vi "IoT Logger Main.vi"() -> ()   [LabVIEW 2019]
uses:
  <vilib>/Utility/miscctls.llb/LVDateTimeRec.ctl
  SubVI/UI/Controls/Pages Tab.ctl
  SubVI/UI/Controls/Home Sensor Heading.ctl
  SubVI/UI/Controls/Buttons/Download Logs.ctl
  SubVI/UI/Controls/Connecting Ring.ctl
  SubVI/UI/Controls/Buttons/Real-time Data.ctl
  SubVI/UI/Controls/Log Row.ctl
  SubVI/UI/Controls/Log Row Download State Indicator.ctl
  SubVI/UI/Controls/Log.ctl
  SubVI/UI/Controls/Log State.ctl
  SubVI/Comms/State Controller/Controls/Comms Loop States.ctl
  SubVI/Messages/Typedefs/Message.ctl
  SubVI/Messages/Typedefs/Sensor Types.ctl
  SubVI/Messages/Typedefs/Message Types.ctl
  SubVI/Application Support/Stop Button/SubVI/Set Stop Button Status.vi
  SubVI/Application Support/Stop Button/SubVI/Get Stop Button Status.vi
  SubVI/Messages/Message Globals.vi
  <userlib>/_OpenG.lib/comparison/comparison.llb/Boolean Changed__ogtk.vi
panel:
  out "Pages":T1
  out "Connecting":T2
  out "Waiting Text":string
  in  "Comissioning":bool
  in  "Real-Time Button":T3
  out "Home Sensor Heading":T4 {"Slide" scale=0.0..100.0; "Free Space" format="%.1f%"}
  in  "Download Button":T5
  out "Log Row 6":T6 {"Download Progress" format="%d%"; "Log Progress" scale=0.0..100.0}
  out "Log Row 5":T6 {"Download Progress" format="%d%"; "Log Progress" scale=0.0..100.0}
  out "Log Row 4":T6 {"Download Progress" format="%d%"; "Log Progress" scale=0.0..100.0}
  out "Log Row 3":T6 {"Download Progress" format="%d%"; "Log Progress" scale=0.0..100.0}
  out "Log Row 2":T6 {"Download Progress" format="%d%"; "Log Progress" scale=0.0..100.0}
  out "Log Row 1":T6 {"Download Progress" format="%d%"; "Log Progress" scale=0.0..100.0}
  out "All Logs Heading":T4 {"Slide" scale=0.0..100.0; "Free Space" format="%.1f%"}
  out "Real-Time Home Heading":T4 {"Slide" scale=0.0..100.0; "Free Space" format="%.1f%"}
  in  "Commissioning Tab":T8(tab)
  in  "Get Log List":bool
  in  "Delete Log File":bool
  in  "Log File to delete":string
  in  "Log File Name":string
  in  "Get Log File":bool
  out "File Size":u32
  in  "Get Log File Size":bool
  out "File Transfer Progress":u32(slide) scale=0.0..54.0
  out "Logs Out":T9[](array[typedef])
  in  "Get SD Card Info":bool
  out "Used SD Card Space (mb)":sgl
  out "Sensor Errors":string[](array[string])
  in  "Send":bool
  in  "Data":u8[](array[numeric])
  in  "Message ID":u8
  in  "Sensor Type":u8
  in  "Payload Length":u8
  out "Turbidity 3":dbl
  out "Turbidity 2":dbl
  out "Turbidity 1":dbl
  out "Turbidity Temp":dbl
  out "Current Measurments":string
  in  "Get Measurements":bool
  in  "Decimal Places":u32=2
  in  "Get RTC Time":bool
  in  "New time":timestamp
  out "Current RTC Time":T11
  out "Logging Period":u32
  in  "Set Logging Period":bool
  in  "Logging Period ms":i32
  in  "Get Logging Period":bool
  out "App Name":string
  in  "Connect":bool
  out "Raw ADC":u32
  out "Battery Voltage":sgl
  in  "Get Battery Info":bool
  in  "Set WiFi Details":bool
  in  "Get WiFi Details":bool
  out "Current WiFi SSID":string
  out "Current WiFi Password":string
  in  "New WiFi Password":string
  in  "New WiFi SSID":string
  out "Heartbeat":bool
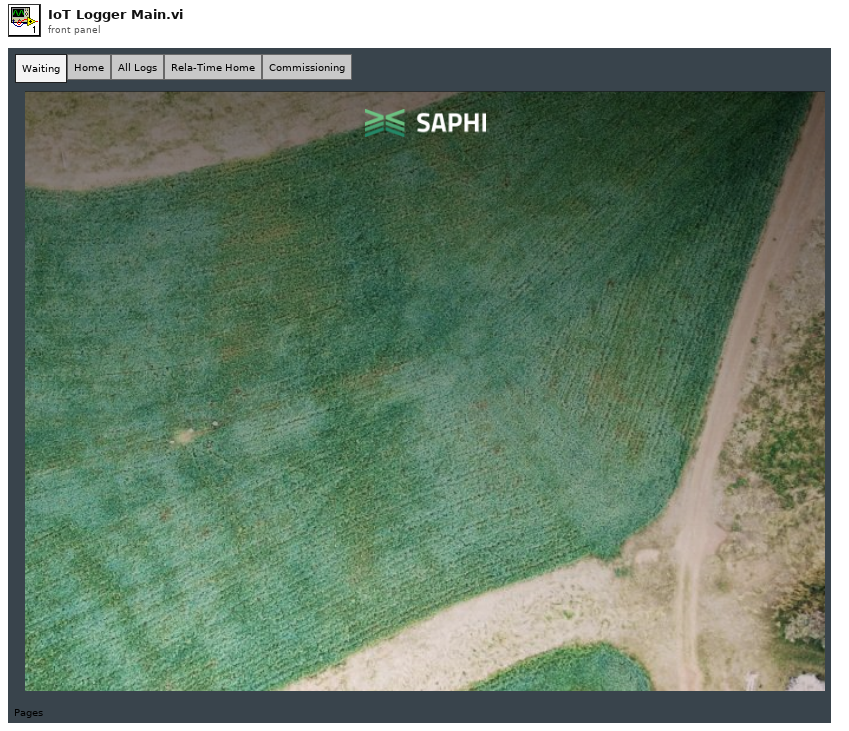
[diagram p1: front panel]
types:
  T1 = typedef "Pages Tab.ctl" = enum32{"Waiting", "Home", "All Logs", "Rela-Time Home", "Commissioning"}
  T2 = typedef "Connecting Ring.ctl" = u16
  T3 = typedef "Real-time Data.ctl" = bool
  T4 = typedef "Home Sensor Heading.ctl" = cluster{"Sensor Name":string, "Free Space":dbl, "Slide":dbl}
  T5 = typedef "Download Logs.ctl" = bool
  T6 = typedef "Log Row.ctl" = cluster{"Day":string, "Date":string, "Log Row Download":T7, "Download Progress":u8, "Log Progress":dbl}
  T7 = typedef "Log Row Download State Indicator.ctl" = u16
  T8 = enum32{"Log Functions", "SD Card Info", "Errors", "Custom Message", "Current Measurements", "RTC", "Logging Period", "Connect", "Batt", "WiFi"}
  T9 = typedef "Log.ctl" = cluster{"Name":string, "Download Percentage":dbl, "Log State":T10}
  T10 = typedef "Log State.ctl" = enum16{"New", "Downloading", "Downloaded"}
  T11 = typedef "LVDateTimeRec.ctl" = cluster{"fractional second":dbl, "second":i32, "minute":i32, "hour":i32, "day of month":i32, "month":i32, "year":i32, "day of week":i32, "day of year":i32, "DST":i32}
  T12 = typedef "Comms Loop States.ctl" = enum16{"Initalise", "User Event", "HEART_BEAT", "SEND_LOG_FILE_NAME", "Clear Log File Names", "SEND_LOG_FILE_CHUNK", "SEND_LOG_FILE_SIZE", "SEND_SD_CARD_INFO", "SEND_BATTERY_INFO", "SEND_LOGGING_PERIOD", "SEND_RTC_TIME", "SEND_CURRENT_MEASUREMENTS", "ERROR_MSG", "Clear Error Messages", "Send Message", "Idle", "Sensor Connected", "Sensor Disconnected", "Set Page Displayed", "Set Connected Sensor Type", "UI: Update Sensor Type", "UI: Update Log List", "Reset Log File Transfer", "SEND_WIFI_DETAILS"}
  T13 = typedef "Message.ctl" = cluster{"Payload Size":u8, "Sequence Number":u8, "Sensor Type":T14, "Message Types":T15, "Data":u8[]}
  T14 = typedef "Sensor Types.ctl" = enum16{"APP", "TURBIDITY", "PH"}
  T15 = typedef "Message Types.ctl" = enum16{"HEART_BEAT", "CONNECT", "GET_CURRENT_MEASUREMENTS", "GET_LOG_FILE", "SEND_LOG_FILE_SIZE", "SEND_LOG_FILE_CHUNK", "GET_LOGGING_PERIOD", "SET_LOGGING_PERIOD", "SEND_SD_CARD_INFO", "GET_LOGS_LIST", "SEND_LOG_FILE_NAME", "SEND_LOGGING_PERIOD", "GET_RTC_TIME", "SET_RTC_TIME", "SEND_RTC_TIME", "SEND_CURRENT_MEASUREMENTS", "DELETE_LOG_FILE", "GET_SD_CARD_INFO", "GET_BATTERY_INFO", "SEND_BATTERY_INFO", "GET_LOG_FILE_SIZE", "SET_WIFI_SSID", "SET_WIFI_PASSWORD", "GET_WIFI_DETAILS", "SEND_WIFI_DETAILS", "ERROR_MSG"}
  T16 = enum16{"open", "replace", "create", "open or create", "replace or create", "replace or create with confirmation"}
  T17 = typedef "eventvkey.ctl" = enum16{"ASCII", "Enter", "Return", "Shift", "Ctrl", "Alt", "Cmd", "Opt", "Caps", "NumLock", "Clear", "Break", "Up", "Down", "Left", "Right", "Insert", "Delete", "Home", "End", "PageUp", "PageDown", "Escape", "Help", "Pause", "ScrollLock", "F1", "F2", "F3", "F4", "F5", "F6", "F7", "F8", "F9", "F10", "F11", "F12", "F13", "F14", "F15", "F16", "F17", "F18", "F19", "F20", "F21", "F22", "F23", "F24", "Play", "VolumeUp", "VolumeDown", "Mute", "Two Byte Char"}
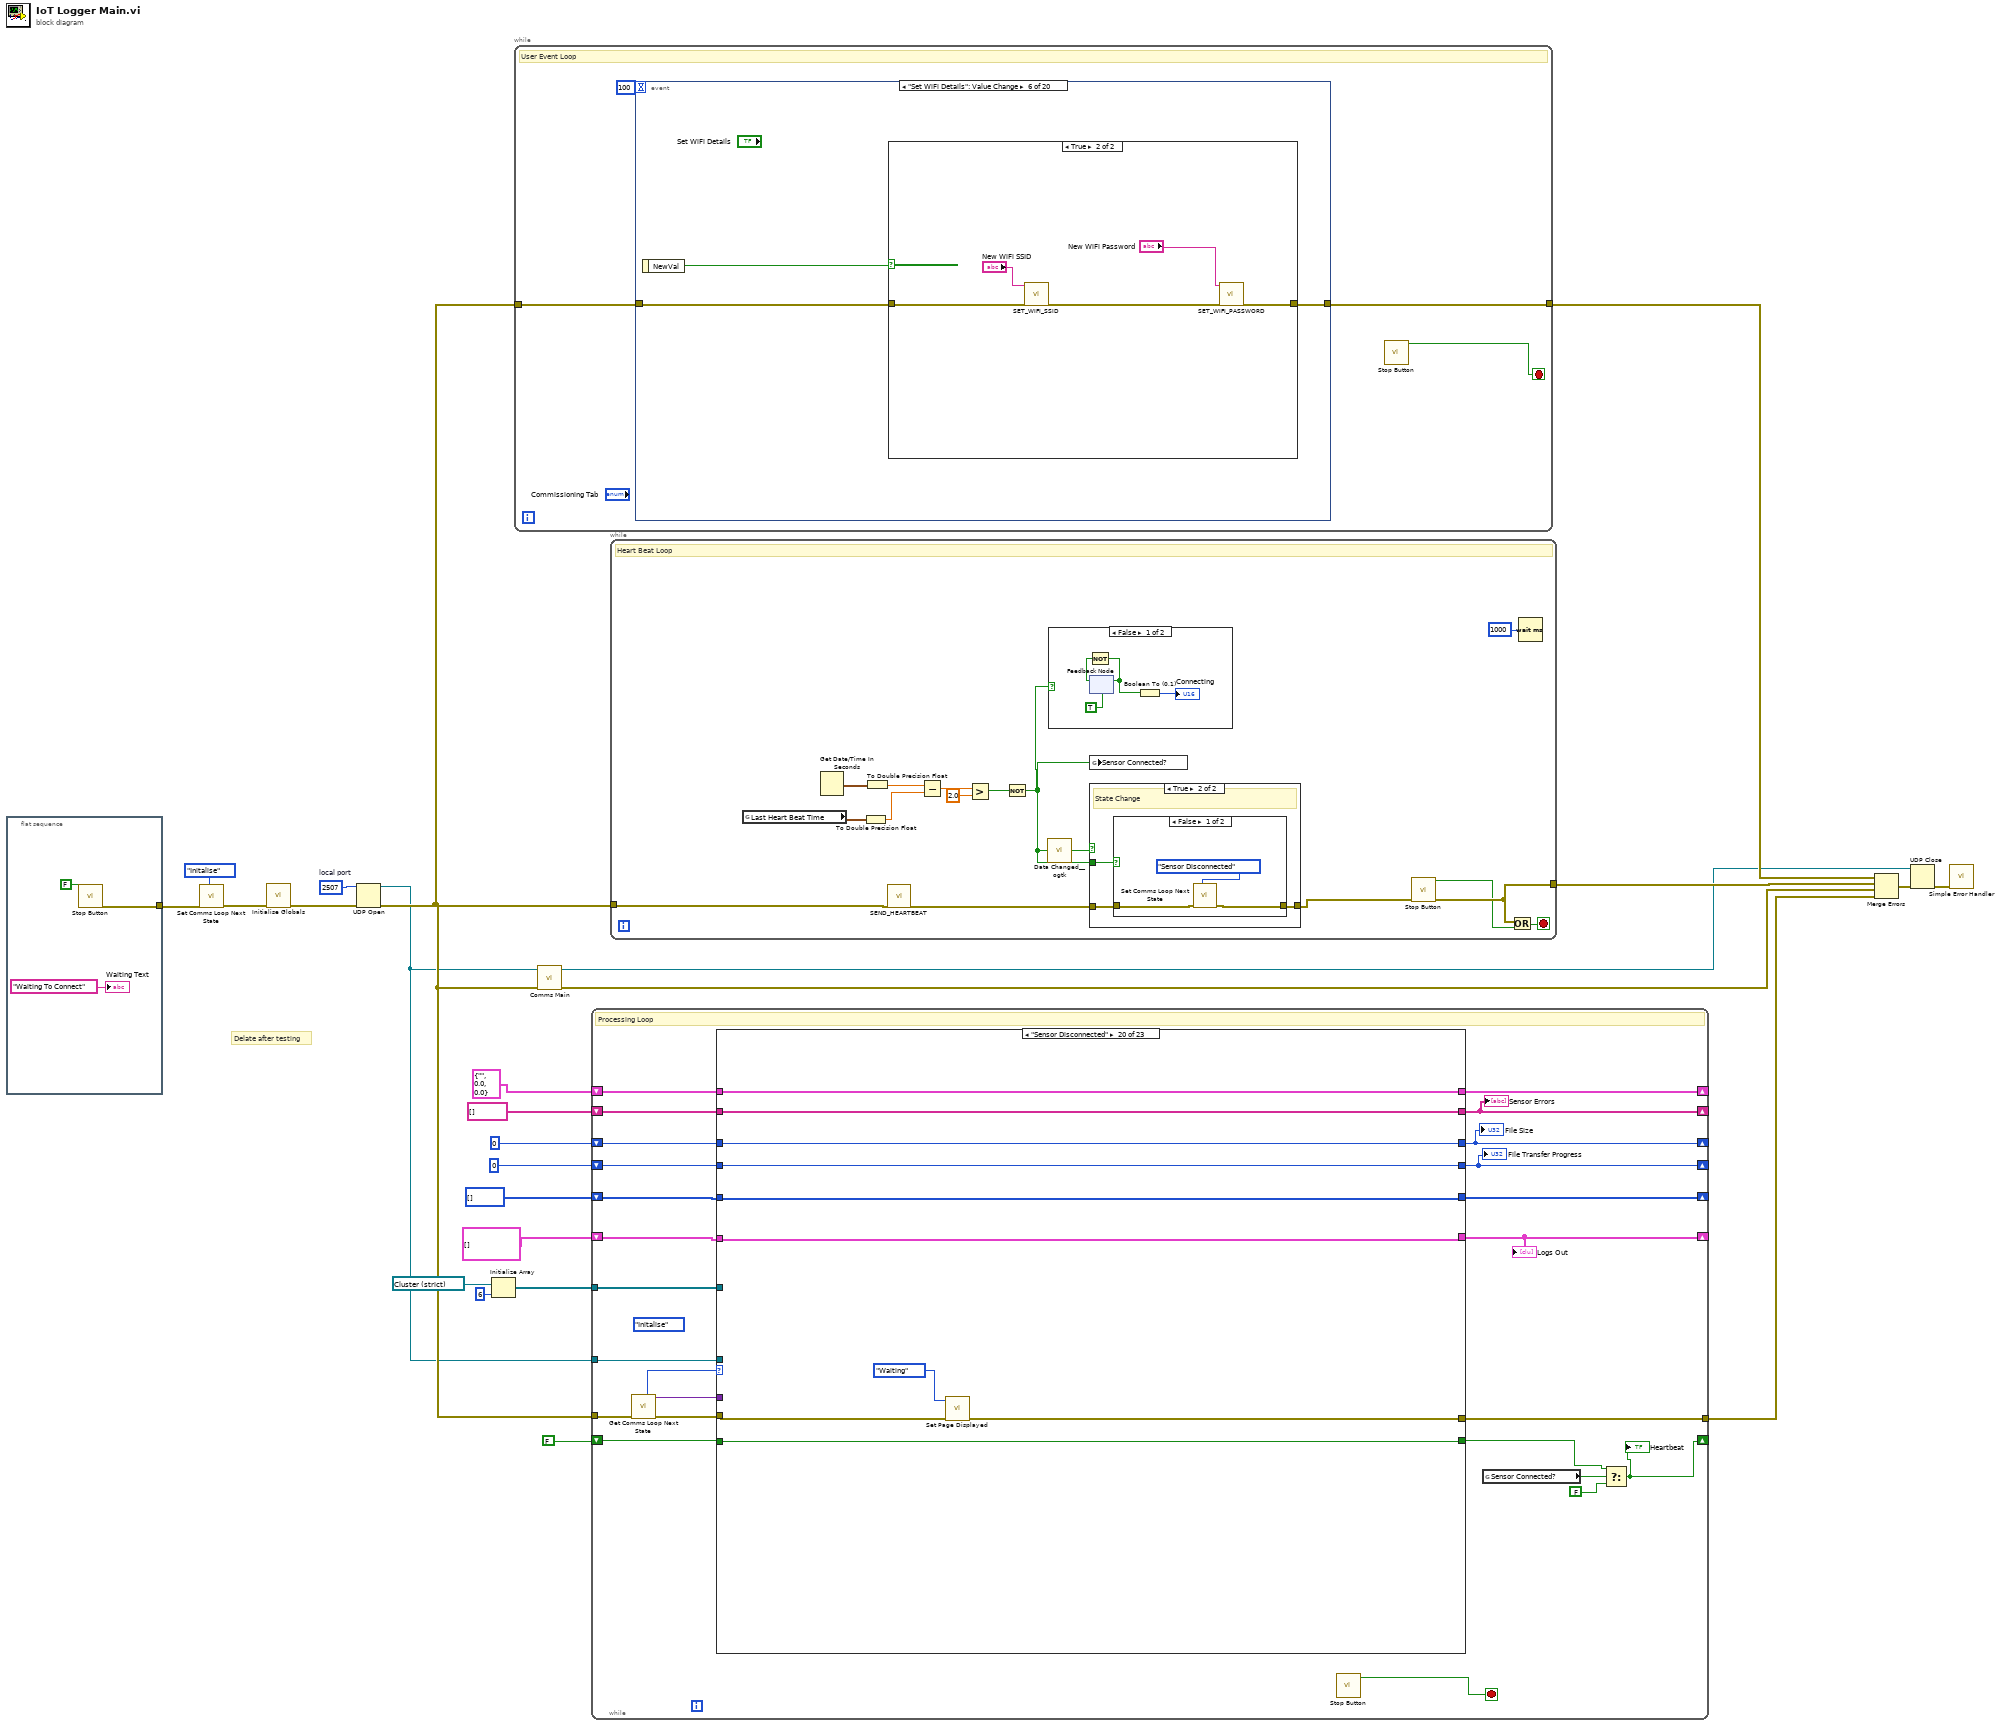
[diagram p0: block diagram]
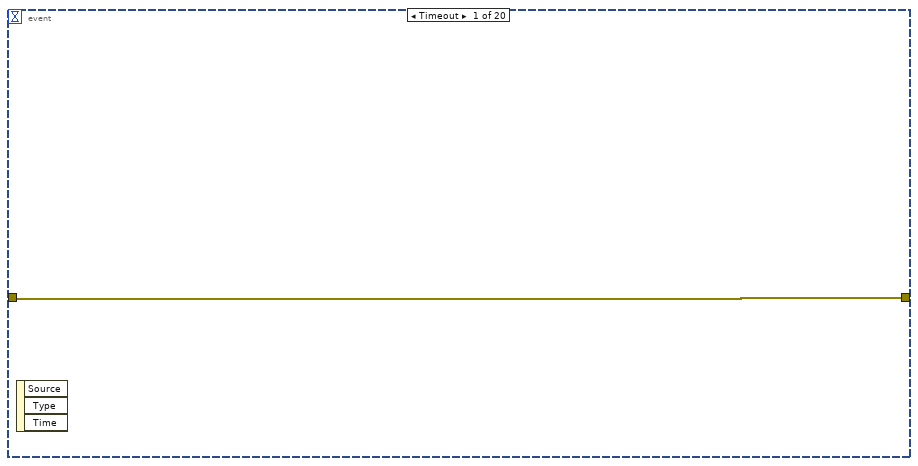
[diagram p2: hidden frame]
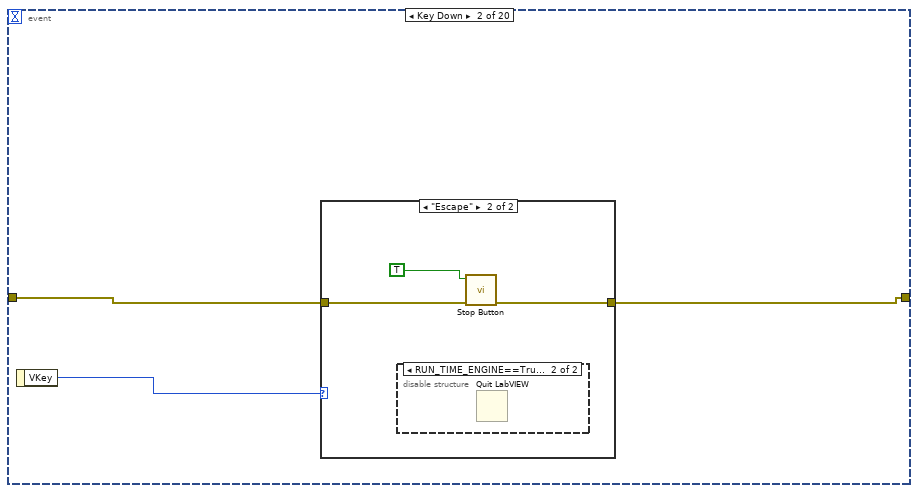
[diagram p3: hidden frame]
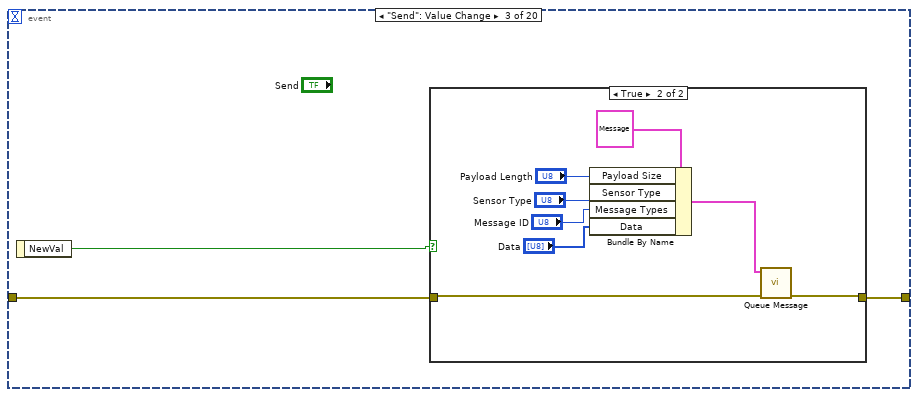
[diagram p6: hidden frame]
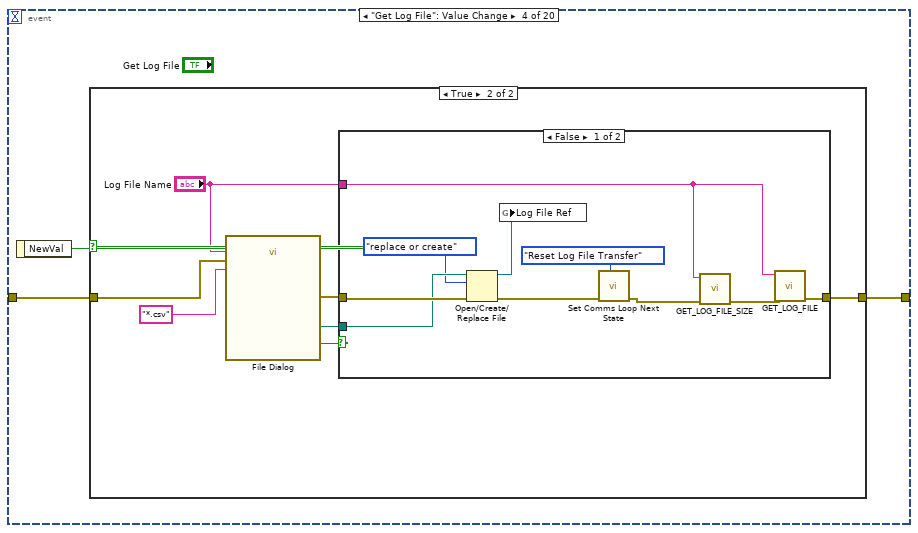
[diagram p8: hidden frame]
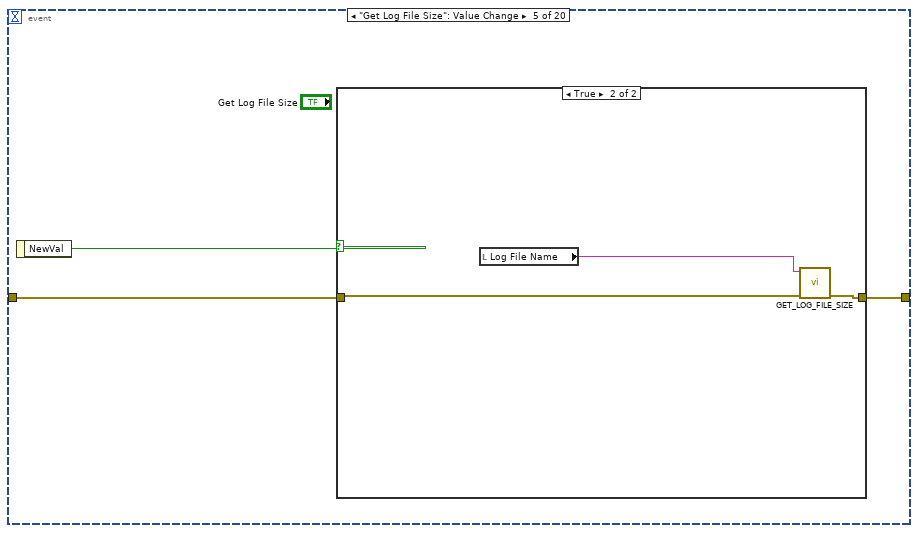
[diagram p11: hidden frame]
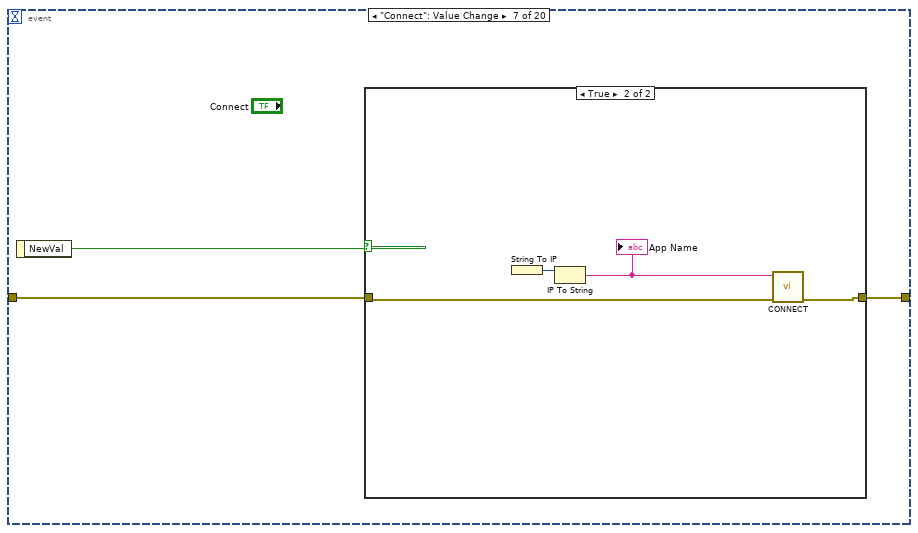
[diagram p14: hidden frame]
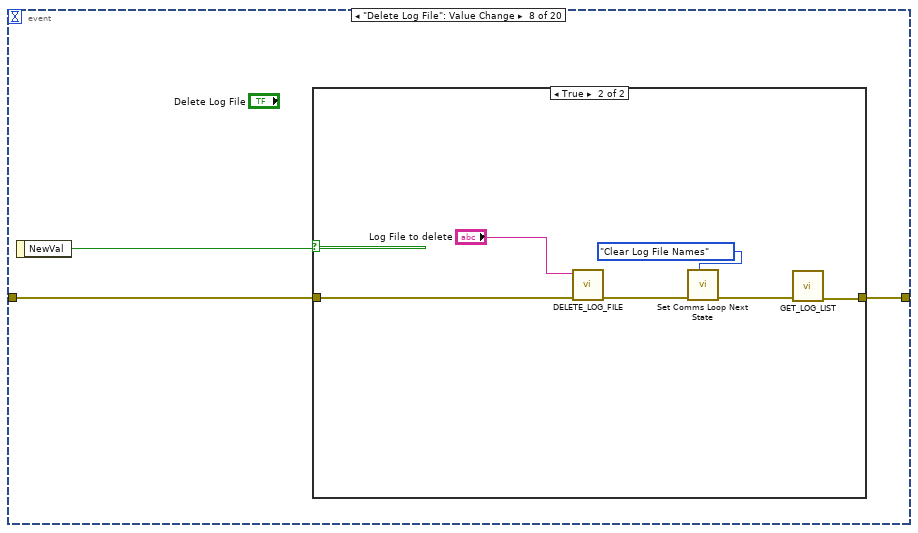
[diagram p16: hidden frame]
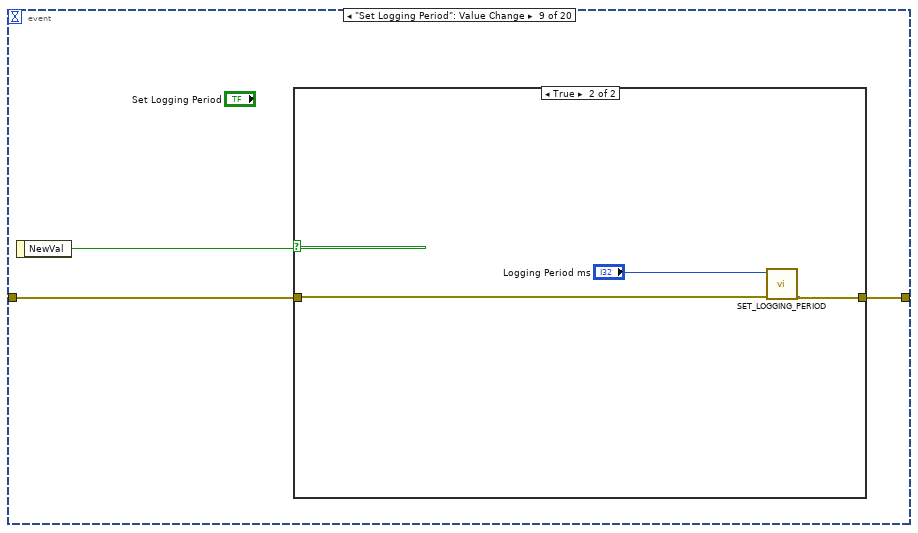
[diagram p18: hidden frame]
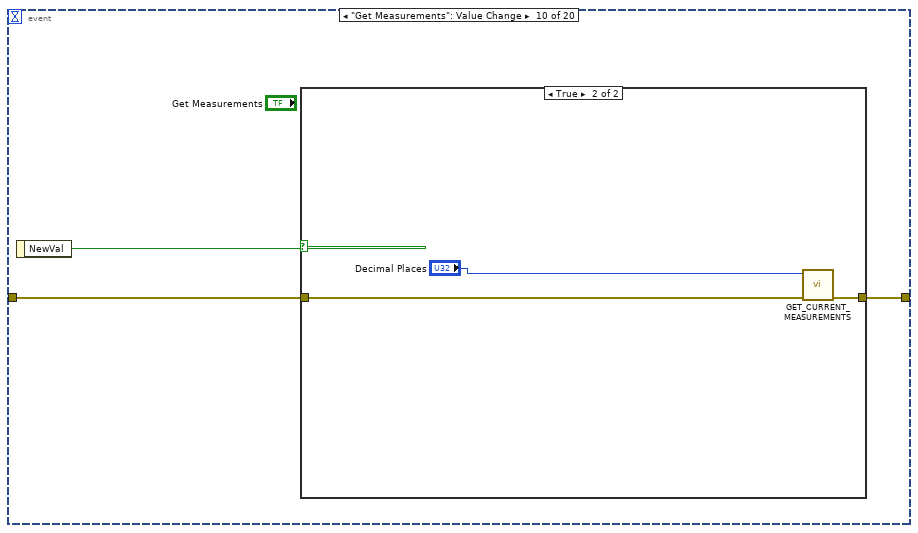
[diagram p20: hidden frame]
diagram:
  w24 = u16 2507  # local port
  # "Delate after testing"
  n1 = flat-sequence {
    tunnel: [w26] -> w5
    frame #0 {
      n2 = call-poly "Stop Button.vi"("Stop Button"=FALSE) -> ("Error Out"=w26:errorcluster)  [unwired: 10 in]
      "Waiting Text" <- "Waiting To Connect" ("Waiting Text")
    }
  }
  n3 = call "Set Comms Loop Next State.vi"("Command"=Comms_Loop_States."Initalise", "error in (no error)"=w5) -> ("error out"=w8:errorcluster)  [unwired: 9 in]
  n4 = call "Initialise Globals.vi"("error in (no error)"=w8) -> ("error out"=w7:errorcluster)  [unwired: 10 in]
  n5 = UDP Open(8:w7, 11:w24) -> (port=w9:refnum<k16>, 0:w19:errorcluster)  [unwired: 3 in, 1 out]
  n6 = Initialize Array(refnum<vi> refnum ("Log Row 1"), 6 ("dimension size")) -> (w2:refnum<vi>[])
  n7 = while {
    tunnel: w19 -> [w30]
    tunnel: [w29] -> w13
    stop <- w31 stop-if-true
    # "User Event Loop"
    n8 = event shown="[5] \"Set WiFi Details\": Value Change" {
      selector: _ -> [_ _ _ _ _ _ _ _ _ _ _ _ _ _ _ _ _ _ _ _]
      dyn-events: _ -> [_ _ _ _ _ _ _ _ _ _ _ _ _ _ _ _ _ _ _ _]
      timeout: 100 -> [_ _ _ _ _ _ _ _ _ _ _ _ _ _ _ _ _ _ _ _]
      tunnel: w30 -> [w32 w34 w41 w53 w75 w82 w91 w99 w109 w116 w123 w129 w135 w141 w147 w155 w161 w165 w168 w171]
      tunnel: [w32 w33 w40 w52 w74 w81 w90 w98 w108 w115 w122 w128 w134 w140 w146 w154 w162 w164 w167 w170] -> w29
      event Timeout {
        n9 = event-data() -> ()  [unwired: 1 in, 3 out]
      }
      event Key Down {
        n10 = event-data() -> ("VKey"=w35:T17)  [unwired: 1 in]
        n11 = case shown="\"Escape\"" w35 {
          tunnel: w34 -> [w36 w38]
          tunnel: [w36 w37] -> w33
          frame "ASCII", Default {
          }
          frame "Escape" {
            n12 = disable-structure shown="RUN_TIME_ENGINE==True" {
              frame condition #0 (active) {
              }
              frame condition #1 {
                n13 = Quit LabVIEW() -> ()  [unwired: 1 in]
              }
            }
            n14 = call-poly "Stop Button.vi"("Error In"=w38, "Stop Button"=TRUE ("Stop Simulator")) -> ("Error Out"=w37:errorcluster)  [unwired: 9 in]
          }
        }
      }
      event "Send": Value Change {
        n15 = event-data() -> ("NewVal"=w42:bool)  [unwired: 1 in]
        n16 = case shown="True" w42 {
          tunnel: w41 -> [w43 w44]
          tunnel: [w43 w51] -> w40
          frame False {
          }
          frame True {
            n17 = Bundle By Name(cluster=T13 {"Payload Size"=0, "Sequence Number"=0, "Sensor Type"=enum."APP", "Message Types"=enum."HEART_BEAT", "Data"=[]} ("Message"), "Payload Size"="Payload Length", "Sensor Type"="Sensor Type", "Message Types"="Message ID", "Data"="Data") -> (w45:T13)
            n18 = call "Queue Message.vi"("error in (no error)"=w44, "Message"=w45) -> ("error out"=w51:errorcluster)  [unwired: 9 in]
          }
        }
      }
      event "Get Log File": Value Change {
        n19 = event-data() -> ("NewVal"=w54:bool)  [unwired: 1 in]
        n20 = case shown="True" w54 {
          tunnel: w53 -> [w55 w61]
          tunnel: [w55 w62] -> w52
          frame False {
          }
          frame True {
            n21 = call "File Dialog"("default name"="Log File Name", "error in"=w61, "pattern (all files)"="*.csv") -> ("selected path"=w59:path, "cancelled"=w60:bool, "error out"=w58:errorcluster)  [unwired: 9 in, 1 out]
            n22 = case shown="False" w60 {
              tunnel: [w68 w73] -> w62
              tunnel: w58 -> [w72 w73]
              tunnel: w59 -> [w71 _]
              tunnel: "Log File Name" -> [w64 _]
              frame False {
                n23 = Open/Create/Replace File(file path (use dialog)=w71, error in=w72, operation (0:open)=T16."replace or create") -> (refnum out=w70:refnum<file>, error out=w67:errorcluster)  [unwired: 3 in, 1 out]
                n24 = global write "Message Globals.vi" "Log File Ref"(w70) -> ()
                n25 = call "Set Comms Loop Next State.vi"("Command"=Comms_Loop_States."Reset Log File Transfer", "error in (no error)"=w67) -> ("error out"=w65:errorcluster)  [unwired: 9 in]
                n26 = call "GET_LOG_FILE_SIZE.vi"("error in (no error)"=w65, "Log File Name"=w64) -> ("error out"=w66:errorcluster)  [unwired: 9 in]
                n27 = call "GET_LOG_FILE.vi"("error in (no error)"=w66, "Log File Name"=w64) -> ("error out"=w68:errorcluster)  [unwired: 9 in]
              }
              frame True {
              }
            }
          }
        }
      }
      event "Get Log File Size": Value Change {
        n28 = event-data() -> ("NewVal"=w76:bool)  [unwired: 1 in]
        n29 = case shown="True" w76 {
          tunnel: w75 -> [w77 w78]
          tunnel: [w77 w80] -> w74
          frame False {
          }
          frame True {
            n30 = local read "Log File Name"() -> (w79:string)
            n31 = call "GET_LOG_FILE_SIZE.vi"("error in (no error)"=w78, "Log File Name"=w79) -> ("error out"=w80:errorcluster)  [unwired: 9 in]
          }
        }
      }
      event "Set WiFi Details": Value Change {
        n32 = event-data() -> ("NewVal"=w83:bool)  [unwired: 1 in]
        n33 = case shown="True" w83 {
          tunnel: w82 -> [w84 w87]
          tunnel: [w84 w89] -> w81
          frame False {
          }
          frame True {
            n34 = call "SET_WIFI_SSID.vi"("error in (no error)"=w87, "New Wifi SSID"="New WiFi SSID") -> ("error out"=w86:errorcluster)  [unwired: 9 in]
            n35 = call "SET_WIFI_PASSWORD.vi"("error in (no error)"=w86, "New Wifi Password"="New WiFi Password") -> ("error out"=w89:errorcluster)  [unwired: 9 in]
          }
        }
      }
      event "Connect": Value Change {
        n36 = event-data() -> ("NewVal"=w92:bool)  [unwired: 1 in]
        n37 = case shown="True" w92 {
          tunnel: w91 -> [w93 w95]
          tunnel: [w93 w96] -> w90
          frame False {
          }
          frame True {
            n38 = String To IP() -> (0:w97:u32)  [unwired: 1 in]
            n39 = IP To String(2:w97) -> (0:w94:string)  [unwired: 1 in]
            "App Name" <- w94
            n40 = call "CONNECT.vi"("error in (no error)"=w95, "Local IP Address"=w94) -> ("error out"=w96:errorcluster)  [unwired: 9 in]
          }
        }
      }
      event "Delete Log File": Value Change {
        n41 = event-data() -> ("NewVal"=w100:bool)  [unwired: 1 in]
        n42 = case shown="True" w100 {
          tunnel: w99 -> [w101 w107]
          tunnel: [w101 w105] -> w98
          frame False {
          }
          frame True {
            n43 = call "DELETE_LOG_FILE.vi"("error in (no error)"=w107, "Log File Name"="Log File to delete") -> ("error out"=w103:errorcluster)  [unwired: 9 in]
            n44 = call "Set Comms Loop Next State.vi"("Command"=Comms_Loop_States."Clear Log File Names", "error in (no error)"=w103) -> ("error out"=w104:errorcluster)  [unwired: 9 in]
            n45 = call "GET_LOG_LIST.vi"("error in (no error)"=w104) -> ("error out"=w105:errorcluster)  [unwired: 10 in]
          }
        }
      }
      event "Set Logging Period": Value Change {
        n46 = event-data() -> ("NewVal"=w110:bool)  [unwired: 1 in]
        n47 = case shown="True" w110 {
          tunnel: w109 -> [w111 w113]
          tunnel: [w111 w114] -> w108
          frame False {
          }
          frame True {
            n48 = call "SET_LOGGING_PERIOD.vi"("error in (no error)"=w113, "Logging Period ms"="Logging Period ms") -> ("error out"=w114:errorcluster)  [unwired: 9 in]
          }
        }
      }
      event "Get Measurements": Value Change {
        n49 = event-data() -> ("NewVal"=w117:bool)  [unwired: 1 in]
        n50 = case shown="True" w117 {
          tunnel: w116 -> [w118 w120]
          tunnel: [w118 w121] -> w115
          frame False {
          }
          frame True {
            n51 = call "GET_CURRENT_MEASUREMENTS.vi"("error in (no error)"=w120, "Decimal Places"="Decimal Places") -> ("error out"=w121:errorcluster)  [unwired: 9 in]
          }
        }
      }
      event "Get Logging Period": Value Change {
        n52 = event-data() -> ("NewVal"=w124:bool)  [unwired: 1 in]
        n53 = case shown="True" w124 {
          tunnel: w123 -> [w125 w126]
          tunnel: [w125 w127] -> w122
          frame False {
          }
          frame True {
            n54 = call "GET_LOGGING_PERIOD.vi"("error in (no error)"=w126) -> ("error out"=w127:errorcluster)  [unwired: 10 in]
          }
        }
      }
      event "Get SD Card Info": Value Change {
        n55 = event-data() -> ("NewVal"=w130:bool)  [unwired: 1 in]
        n56 = case shown="True" w130 {
          tunnel: w129 -> [w131 w132]
          tunnel: [w131 w133] -> w128
          frame False {
          }
          frame True {
            n57 = call "GET_SD_CARD_INFO.vi"("error in (no error)"=w132) -> ("error out"=w133:errorcluster)  [unwired: 10 in]
          }
        }
      }
      event "Get WiFi Details": Value Change {
        n58 = event-data() -> ("NewVal"=w136:bool)  [unwired: 1 in]
        n59 = case shown="True" w136 {
          tunnel: w135 -> [w137 w138]
          tunnel: [w137 w139] -> w134
          frame False {
          }
          frame True {
            n60 = call "GET_WIFI_DETAILS.vi"("error in (no error)"=w138) -> ("error out"=w139:errorcluster)  [unwired: 10 in]
          }
        }
      }
      event "Get Battery Info": Value Change {
        n61 = event-data() -> ("NewVal"=w142:bool)  [unwired: 1 in]
        n62 = case shown="True" w142 {
          tunnel: w141 -> [w143 w144]
          tunnel: [w143 w145] -> w140
          frame False {
          }
          frame True {
            n63 = call "GET_BATTERY_INFO.vi"("error in (no error)"=w144) -> ("error out"=w145:errorcluster)  [unwired: 10 in]
          }
        }
      }
      event "Get Log List": Value Change {
        n64 = event-data() -> ("NewVal"=w148:bool)  [unwired: 1 in]
        n65 = case shown="True" w148 {
          tunnel: w147 -> [w149 w151]
          tunnel: [w149 w153] -> w146
          frame False {
          }
          frame True {
            n66 = call "Set Comms Loop Next State.vi"("Command"=Comms_Loop_States."Clear Log File Names", "error in (no error)"=w151) -> ("error out"=w152:errorcluster)  [unwired: 9 in]
            n67 = call "GET_LOG_LIST.vi"("error in (no error)"=w152) -> ("error out"=w153:errorcluster)  [unwired: 10 in]
          }
        }
      }
      event "Get RTC Time": Value Change {
        n68 = event-data() -> ("NewVal"=w156:bool)  [unwired: 1 in]
        n69 = case shown="True" w156 {
          tunnel: w155 -> [w157 w158]
          tunnel: [w157 w159] -> w154
          frame False {
          }
          frame True {
            n70 = call "GET_RTC_TIME.vi"("error in (no error)"=w158) -> ("error out"=w159:errorcluster)  [unwired: 10 in]
          }
        }
      }
      event "New time": Value Change {
        n71 = event-data() -> ("NewVal"=w160:timestamp)  [unwired: 1 in]
        n72 = call "SET_RTC_TIME.vi"("error in (no error)"=w161, "New Time"=w160) -> ("error out"=w162:errorcluster)  [unwired: 9 in]
      }
      event Value Change {
        n73 = event-data() -> ()  [unwired: 1 in, 6 out]
        n74 = call "Set Page Displayed.vi"("error in (no error)"=w165, "Page to display"=Pages_Tab."All Logs") -> ("error out"=w164:errorcluster)  [unwired: 9 in]
      }
      event Value Change {
        n75 = event-data() -> ()  [unwired: 1 in, 6 out]
        n76 = call "Set Page Displayed.vi"("error in (no error)"=w168, "Page to display"=Pages_Tab."Rela-Time Home") -> ("error out"=w167:errorcluster)  [unwired: 9 in]
      }
      event "Comissioning": Value Change {
        n77 = event-data() -> ()  [unwired: 1 in, 6 out]
        n78 = call "Set Page Displayed.vi"("error in (no error)"=w171, "Page to display"=Pages_Tab."Commissioning") -> ("error out"=w170:errorcluster)  [unwired: 9 in]
      }
    }
    n79 = call-poly "Stop Button.vi"() -> ("Stop ButtonOut"=w31:bool)  [unwired: 10 in, 1 out]
  }
  n80 = call "Comms Main.vi"("error in (no error)"=w19, "UDP Ref"=w9) -> ("error out"=w12:errorcluster, "UDP Ref Out"=w11:refnum<k16>)  [unwired: 8 in]
  n81 = while {
    tunnel: w19 -> [w195]
    shift-right: [w190] -> _
    shift-left: T9[] [] -> [w191]
    shift-right: [w188] -> _
    shift-left: u8[] [] ("Log File Chunk") -> [w189]
    shift-right: [w182] -> _
    shift-left: u32 0 -> [w187]
    shift-right: [w185] -> _
    shift-left: u32 0 -> [w186]
    shift-right: [w183] -> _
    shift-left: string[] [] -> [w184]
    tunnel: [w181] -> w10
    tunnel: w9 -> [w180]
    shift-right: [w178] -> _
    shift-left: T4 {"Sensor Name"="", "Free Space"=0.0, "Slide"=0.0} ("Home Sensor Heading") -> [w179]
    tunnel: w2 -> [w177]
    shift-right: [w172] -> _
    shift-left: FALSE -> [w176]
    stop <- w196 stop-if-true
    (unwired) Comms_Loop_States."Initalise" ("Command")
    # "Processing Loop"
    n82 = call "Get Comms Loop Next State.vi"("error in (no error)"=w195) -> ("error out"=w194:errorcluster, "Data"=w192:variant, "Command"=w193:T12)  [unwired: 8 in]
    n83 = case shown="\"Sensor Disconnected\"" w193 {
      tunnel: w194 -> [w201 w223 w250 w254 w263 w285 w305 w323 w338 w352 w366 w382 w404 w425 w433 w447 w455 w472 w486 w493 w508 w516 w526]
      tunnel: w192 -> [_ w222 w249 _ _ w284 w306 w324 w339 w353 w367 w383 w405 w424 _ w446 _ _ w485 _ w507 _ _]
      tunnel: w191 -> [_ w220 w240 _ w266 w286 w310 w329 w344 w358 w372 w388 w415 w430 w438 w452 w460 w477 w491 w501 w513 w521 w524]
      tunnel: [T9[] [] ("Logs Out") w220 w238 T9[] [] ("Logs Out") w266 w286 w310 w329 w344 w358 w372 w388 w415 w430 w438 w452 w460 w477 w491 w501 w513 w521 w524] -> w190
      tunnel: w189 -> [_ w216 w245 w258 _ w280 w309 w328 w343 w357 w371 w387 w414 w429 w437 w451 w459 w476 w490 w500 w512 w520 w539]
      tunnel: [u8[] [] ("Log File Chunk") w216 w245 w258 u8[] [] ("Log File Chunk") w268 w309 w328 w343 w357 w371 w387 w414 w429 w437 w451 w459 w476 w490 w500 w512 w520 w539] -> w188
      tunnel: w187 -> [_ w215 w244 w257 _ w278 w308 w327 w342 w356 w370 w386 w413 w428 w436 w450 w458 w475 w489 w499 w511 w519 w538]
      tunnel: [u32 0 w215 w244 w257 u32 0 w276 w308 w327 w342 w356 w370 w386 w413 w428 w436 w450 w458 w475 w489 w499 w511 w519 w538] -> w182
      tunnel: w186 -> [_ w214 w243 w256 w265 w275 _ w326 w341 w355 w369 w385 w412 w427 w435 w449 w457 w474 w488 w498 w510 w518 w537]
      tunnel: [u32 0 ("Log File Size") w214 w243 w256 w265 w275 w301 w326 w341 w355 w369 w385 w412 w427 w435 w449 w457 w474 w488 w498 w510 w518 w537] -> w185
      tunnel: w184 -> [_ w213 w242 w255 w264 w272 w300 w320 w333 w348 w362 w376 w411 w421 _ w448 w456 w473 w487 w497 w509 w517 w536]
      tunnel: [string[] [] w213 w242 w255 w264 w272 w300 w320 w333 w348 w362 w376 w411 w419 string[] [] w448 w456 w473 w487 w497 w509 w517 w536] -> w183
      tunnel: [w199 w212 w237 w254 w263 w271 w299 w319 w332 w347 w361 w375 w401 w418 w433 w442 w455 w465 w479 w492 w504 w516 w525] -> w181
      tunnel: w180 -> [_ _ _ _ _ _ _ _ _ _ _ _ _ _ _ w441 _ _ _ _ _ _ _]
      tunnel: w179 -> [_ w211 w241 w253 w262 w270 w298 w316 w331 w346 w360 w374 w410 w417 w432 w440 w454 w464 w483 w496 w503 w515 w535]
      tunnel: [T4 {"Sensor Name"="", "Free Space"=0.0, "Slide"=0.0} ("Home Sensor Heading") w211 w241 w253 w262 w270 w298 w315 w331 w346 w360 w374 w410 w417 w432 w440 w454 w464 w480 w496 w503 w515 w535] -> w178
      tunnel: w177 -> [_ _ _ _ _ _ _ _ _ _ _ _ _ _ _ _ _ _ _ _ _ _ w528]
      tunnel: w176 -> [w197 w208 w233 w251 w259 w267 w297 w311 w330 w345 w359 w373 w409 w416 w431 w439 w453 w463 w478 w495 w502 w514 w522]
      tunnel: [w197 w207 w233 w251 w259 w267 w297 w311 w330 w345 w359 w373 w409 w416 w431 w439 w453 w463 w478 w495 w502 w514 w522] -> w174
      frame "Initalise" {
        (unwired) T9[] [{"Name"="21-02-14.csv", "Download Percentage"=0.0, "Log State"=enum."New"}, {"Name"="21-02-15.csv", "Download Percentage"=0.0, "Log State"=enum."New"}, {"Name"="21-02-16.csv", "Download Percentage"=0.0, "Log State"=enum."New"}, {"Name"="21-02-17.csv", "Download Percentage"=0.0, "Log State"=enum."New"}, {"Name"="21-02-18.csv", "Download Percentage"=0.0, "Log State"=enum."New"}, {"Name"="21-02-19.csv", "Download Percentage"=0.0, "Log State"=enum."New"}] ("Logs Out")
        n84 = call "Set Comms Loop Next State.vi"("Command"=Comms_Loop_States."UI: Update Log List", "error in (no error)"=w201) -> ("error out"=w199:errorcluster)  [unwired: 9 in]
      }
      frame "HEART_BEAT" {
        n85 = Variant To Data(error in=w223, type=T13 {"Payload Size"=0, "Sequence Number"=0, "Sensor Type"=enum."APP", "Message Types"=enum."SEND_LOG_FILE_SIZE", "Data"=[]} ("Message"), Variant=w222) -> (data=w210:T13, error out=w217:errorcluster)
        n86 = Unbundle By Name(w210) -> ("Sensor Type"=w209:T14)
        n87 = call "HEART_BEAT.vi"("error in (no error)"=w217, "Message"=w210) -> ("error out"=w218:errorcluster, "HB Good?"=w219:bool)  [unwired: 8 in]
        n88 = case shown="False" w219 {
          tunnel: [w225 w230] -> w212
          tunnel: w218 -> [w225 w229]
          tunnel: w209 -> [_ w228]
          tunnel: w208 -> [w224 w227]
          tunnel: [w224 w226] -> w207
          frame False {
            # "Bad Heart beat, do nothing"
          }
          frame True {
            # "Heart beat good, reset timer"
            n89 = Get Date/Time In Seconds() -> (seconds since 1Jan1904=w232:timestamp)
            n90 = call "Set Comms Loop Next State.vi"("Command"=Comms_Loop_States."Set Connected Sensor Type", "error in (no error)"=w229, "Data"=w228) -> ("error out"=w230:errorcluster)  [unwired: 8 in]
            n91 = Not(x=w227) -> (.not. x?=w226:bool)
            n92 = global write "Message Globals.vi" "Last Heart Beat Time"(w232) -> ()
          }
        }
      }
      frame "SEND_LOG_FILE_NAME" {
        n93 = Variant To Data(error in=w250, type=T13 {"Payload Size"=0, "Sequence Number"=0, "Sensor Type"=enum."APP", "Message Types"=enum."SEND_LOG_FILE_SIZE", "Data"=[]} ("Message"), Variant=w249) -> (data=w247:T13, error out=w246:errorcluster)
        n94 = call "SEND_LOG_FILE_NAME.vi"("error in (no error)"=w246, "Message"=w247) -> ("error out"=w239:errorcluster, "Log File Name"=w234:string)  [unwired: 8 in]
        n95 = Bundle By Name(cluster=T9 {"Name"="", "Download Percentage"=0.0, "Log State"=enum."New"} ("New Log"), "Name"=w234) -> (w235:T9)
        n96 = call "Add Log File.vi"("error in (no error)"=w239, "New Log"=w235, "Logs"=w240) -> ("error out"=w237:errorcluster, "Logs Out"=w238:T9[])  [unwired: 7 in]
      }
      frame "Clear Log File Names" {
      }
      frame "Reset Log File Transfer" {
      }
      frame "SEND_LOG_FILE_CHUNK" {
        n97 = Variant To Data(error in=w285, type=T13 {"Payload Size"=0, "Sequence Number"=0, "Sensor Type"=enum."APP", "Message Types"=enum."SEND_LOG_FILE_SIZE", "Data"=[]} ("Message"), Variant=w284) -> (data=w281:T13, error out=w282:errorcluster)
        n98 = call "SEND_LOG_FILE_CHUNK.vi"("error in (no error)"=w282, "Message"=w281) -> ("error out"=w273:errorcluster, "Chunk Size"=w277:i32, "Log File Chunk"=w279:u8[])  [unwired: 7 in]
        n99 = Build Array (concatenate)(w280, w279) -> (w269:u8[])
        n100 = Add(x=w278, y=w277) -> (x+y=w276:u32)
        n101 = Greater Or Equal?(x=w276, y=w275) -> (x >= y?=w274:bool)
        n102 = case shown="True" w274 {
          tunnel: w273 -> [w288 w295]
          tunnel: [w288 w290] -> w271
          tunnel: w269 -> [w287 w294]
          tunnel: [w287 u8[] []] -> w268
          frame False {
            # "Still Recieving log file bytes so update progress"
          }
          frame True {
            # "All bytes recieved, process log file"
            n103 = Byte Array To String(unsigned byte array=w294) -> (string=w293:string)
            n104 = global read "Message Globals.vi" "Log File Ref"() -> (w296:refnum<file>)
            n105 = Write to Text File(file (use dialog)=w296, text=w293, error in=w295) -> (refnum out=w292:refnum<file>, error out=w291:errorcluster)  [unwired: 1 in, 1 out]
            n106 = Close File(refnum=w292, error in=w291) -> (error out=w290:errorcluster)  [unwired: 1 out]
          }
        }
      }
      frame "SEND_LOG_FILE_SIZE" {
        n107 = Variant To Data(error in=w305, type=T13 {"Payload Size"=0, "Sequence Number"=0, "Sensor Type"=enum."APP", "Message Types"=enum."SEND_LOG_FILE_SIZE", "Data"=[]} ("Message"), Variant=w306) -> (data=w304:T13, error out=w303:errorcluster)
        n108 = call "SEND_LOG_FILE_SIZE.vi"("error in (no error)"=w303, "Message"=w304) -> ("error out"=w302:errorcluster, "Log File Size"=w301:u32)  [unwired: 8 in]
        n109 = property on="File Transfer Progress" class="Slide (strict)"(error in=w302, "Scale.Maximum"=w301) -> (error out=w299:errorcluster)  [unwired: 1 in, 1 out]
      }
      frame "SEND_SD_CARD_INFO" {
        # "mb in a 32gb SD card"
        n110 = Variant To Data(error in=w323, type=T13 {"Payload Size"=0, "Sequence Number"=0, "Sensor Type"=enum."APP", "Message Types"=enum."SEND_LOG_FILE_SIZE", "Data"=[]} ("Message"), Variant=w324) -> (data=w321:T13, error out=w322:errorcluster)
        n111 = call "SEND_SD_CARD_INFO.vi"("error in (no error)"=w322, "Message"=w321) -> ("error out"=w319:errorcluster, "Used Space (mb)"=w318:sgl)  [unwired: 8 in]
        "Used SD Card Space (mb)" <- w318
        n112 = Divide(x=w318, y=sgl 27464.0) -> (x/y=w314:sgl)
        n113 = Multiply(x=sgl 100.0, y=w314) -> (x*y=w312:sgl)
        n114 = Bundle By Name(cluster=w316, "Free Space"=w312, "Slide"=w312) -> (w315:T4)
      }
      frame "SEND_BATTERY_INFO" {
        n115 = Variant To Data(error in=w338, type=T13 {"Payload Size"=0, "Sequence Number"=0, "Sensor Type"=enum."APP", "Message Types"=enum."SEND_LOG_FILE_SIZE", "Data"=[]} ("Message"), Variant=w339) -> (data=w336:T13, error out=w337:errorcluster)
        n116 = call "SEND_BATTERY_INFO.vi"("error in (no error)"=w337, "Message"=w336) -> ("error out"=w332:errorcluster, "Raw ADC"=→"Raw ADC":u32, "Battery Voltage"=→"Battery Voltage":sgl)  [unwired: 7 in]
      }
      frame "SEND_LOGGING_PERIOD" {
        n117 = Variant To Data(error in=w352, type=T13 {"Payload Size"=0, "Sequence Number"=0, "Sensor Type"=enum."APP", "Message Types"=enum."SEND_LOG_FILE_SIZE", "Data"=[]} ("Message"), Variant=w353) -> (data=w350:T13, error out=w351:errorcluster)
        n118 = call "SEND_LOGGING_PERIOD.vi"("error in (no error)"=w351, "Message"=w350) -> ("error out"=w347:errorcluster, "Logging Period"=→"Logging Period":u32)  [unwired: 8 in]
      }
      frame "SEND_RTC_TIME" {
        n119 = Variant To Data(error in=w366, type=T13 {"Payload Size"=0, "Sequence Number"=0, "Sensor Type"=enum."APP", "Message Types"=enum."SEND_LOG_FILE_SIZE", "Data"=[]} ("Message"), Variant=w367) -> (data=w364:T13, error out=w365:errorcluster)
        n120 = call "SEND_RTC_TIME.vi"("error in (no error)"=w365, "Message"=w364) -> ("error out"=w361:errorcluster, "Current RTC Time"=→"Current RTC Time":T11)  [unwired: 8 in]
      }
      frame "SEND_CURRENT_MEASUREMENTS" {
        n121 = Variant To Data(error in=w382, type=T13 {"Payload Size"=0, "Sequence Number"=0, "Sensor Type"=enum."APP", "Message Types"=enum."SEND_LOG_FILE_SIZE", "Data"=[]} ("Message"), Variant=w383) -> (data=w380:T13, error out=w381:errorcluster)
        n122 = call "SEND_CURRENT_MEASUREMENTS.vi"("error in (no error)"=w381, "Message"=w380) -> ("error out"=w378:errorcluster, "Current Measurments (csv string)"=w377:string)  [unwired: 8 in]
        "Current Measurments" <- w377
        n123 = Unbundle By Name(w380) -> ("Sensor Type"=w379:T14)
        n124 = case shown="\"TURBIDITY\"" w379 {
          tunnel: w378 -> [w389 w390]
          tunnel: w377 -> [_ w399]
          tunnel: [w389 w390] -> w375
          frame "APP", Default {
          }
          frame "TURBIDITY" {
            n125 = Spreadsheet String To Array(delimiter (Tab)=",", format string="%f", spreadsheet string=w399, array type (2D Dbl)=dbl[] []) -> (array=w397:dbl[])
            n126 = Index Array(array=w397, index #1=0 ("index")) -> (element #1=→"Turbidity Temp":dbl, element #2=→"Turbidity 1":dbl, element #3=→"Turbidity 2":dbl, element #4=→"Turbidity 3":dbl)  [unwired: 3 in]
          }
        }
      }
      frame "SEND_WIFI_DETAILS" {
        n127 = Variant To Data(error in=w404, type=T13 {"Payload Size"=0, "Sequence Number"=0, "Sensor Type"=enum."APP", "Message Types"=enum."SEND_LOG_FILE_SIZE", "Data"=[]} ("Message"), Variant=w405) -> (data=w406:T13, error out=w407:errorcluster)
        n128 = call "SEND_WIFI_DETAILS.vi"("error in (no error)"=w407, "Message"=w406) -> ("error out"=w401:errorcluster, "Password"=→"Current WiFi Password":string, "SSID"=→"Current WiFi SSID":string)  [unwired: 7 in]
      }
      frame "ERROR_MSG" {
        n129 = Variant To Data(error in=w425, type=T13 {"Payload Size"=0, "Sequence Number"=0, "Sensor Type"=enum."APP", "Message Types"=enum."SEND_LOG_FILE_SIZE", "Data"=[]} ("Message"), Variant=w424) -> (data=w422:T13, error out=w423:errorcluster)
        n130 = call "ERROR_MSG.vi"("error in (no error)"=w423, "Message"=w422) -> ("error out"=w418:errorcluster, "Error Msg String"=w420:string)  [unwired: 8 in]
        n131 = Build Array (concatenate)(w420, w421) -> (w419:string[])
      }
      frame "Clear Error Messages" {
      }
      frame "Send Message" {
        n132 = Variant To Data(error in=w447, type=T13 {"Payload Size"=0, "Sequence Number"=0, "Sensor Type"=enum."APP", "Message Types"=enum."HEART_BEAT", "Data"=[]} ("Message"), Variant=w446) -> (data=w443:T13, error out=w444:errorcluster)
        n133 = call "Send Message.vi"("error in (no error)"=w444, "Message"=w443, "UDP Ref"=w441) -> ("error out"=w442:errorcluster)  [unwired: 7 in, 1 out]
      }
      frame "Idle", Default {
        "Real-Time Home Heading" <- w454
        "Home Sensor Heading" <- w454
        "All Logs Heading" <- w454
      }
      frame "Sensor Connected" {
        n134 = String To IP() -> (0:w468:u32)  [unwired: 1 in]
        n135 = IP To String(2:w468) -> (0:w467:string)  [unwired: 1 in]
        n136 = call "CONNECT.vi"("error in (no error)"=w472, "Local IP Address"=w467) -> ("error out"=w471:errorcluster)  [unwired: 9 in]
        n137 = call "GET_LOG_LIST.vi"("error in (no error)"=w471) -> ("error out"=w470:errorcluster)  [unwired: 10 in]
        n138 = call "GET_SD_CARD_INFO.vi"("error in (no error)"=w470) -> ("error out"=w469:errorcluster)  [unwired: 10 in]
        n139 = call "GET_RTC_TIME.vi"("error in (no error)"=w469) -> ("error out"=w462:errorcluster)  [unwired: 10 in]
        n140 = call "GET_WIFI_DETAILS.vi"("error in (no error)"=w462) -> ("error out"=w461:errorcluster)  [unwired: 10 in]
        n141 = call "Set Page Displayed.vi"("error in (no error)"=w461, "Page to display"=Pages_Tab."Home") -> ("error out"=w465:errorcluster)  [unwired: 9 in]
      }
      frame "Set Connected Sensor Type" {
        n142 = Variant To Data(error in=w486, type=Sensor_Types."APP" ("Sensor Type"), Variant=w485) -> (data=w482:T14, error out=w479:errorcluster)
        n143 = global write "Message Globals.vi" "Connected Sensor Type"(w482) -> ()
        n144 = call "Sensor Type to String.vi"("Sensor Type"=w482) -> ("Sensor String"=w481:string)  [unwired: 10 in]
        n145 = Bundle By Name(cluster=w483, "Sensor Name"=w481) -> (w480:T4)
      }
      frame "Sensor Disconnected" {
        n146 = call "Set Page Displayed.vi"("error in (no error)"=w493, "Page to display"=Pages_Tab."Waiting") -> ("error out"=w492:errorcluster)  [unwired: 9 in]
      }
      frame "Set Page Displayed" {
        n147 = Variant To Data(error in=w508, type=Pages_Tab."Home" ("Pages"), Variant=w507) -> (data=w505:T1, error out=w504:errorcluster)
        "Pages" <- w505
        n148 = global write "Message Globals.vi" "Pages"(w505) -> ()
      }
      frame "UI: Update Sensor Type" {
      }
      frame "UI: Update Log List" {
        n149 = control-ref of="Log Row 1"() -> (w534:refnum<vi>)
        n150 = control-ref of="Log Row 2"() -> (w533:refnum<vi>)
        n151 = control-ref of="Log Row 3"() -> (w532:refnum<vi>)
        n152 = control-ref of="Log Row 4"() -> (w531:refnum<vi>)
        n153 = control-ref of="Log Row 5"() -> (w530:refnum<vi>)
        n154 = control-ref of="Log Row 6"() -> (w529:refnum<vi>)
        n155 = Insert Into Array(array=w528, index=0, new element #1=w534, new element #2=w533, new element #3=w532, new element #4=w531, new element #5=w530, new element #6=w529) -> (w523:refnum<vi>[])
        n156 = call "Update UI Logs Display.vi"("error in (no error)"=w526, "Display References"=w523, "Log Array Subset"=w524) -> ("error out"=w525:errorcluster)  [unwired: 8 in]
      }
    }
    "File Size" <- w185
    "Sensor Errors" <- w183
    "File Transfer Progress" <- w182
    "Logs Out" <- w190
    n157 = call-poly "Stop Button.vi"() -> ("Stop ButtonOut"=w196:bool)  [unwired: 10 in, 1 out]
    n158 = global read "Message Globals.vi" "Sensor Connected?"() -> (w175:bool)
    n159 = Select(t=w174, s=w175, f=FALSE) -> (s? t:f=w172:bool)
    "Heartbeat" <- w172
  }
  n160 = while {
    tunnel: w19 -> [w545]
    tunnel: [w546] -> w22
    stop <- w555 stop-if-true
    # "Heart Beat Loop"
    n161 = global read "Message Globals.vi" "Last Heart Beat Time"() -> (w552:timestamp)
    n162 = Get Date/Time In Seconds() -> (seconds since 1Jan1904=w553:timestamp)
    n163 = To Double Precision Float(number=w552) -> (double precision float=w550:dbl)
    n164 = To Double Precision Float(number=w553) -> (double precision float=w551:dbl)
    n165 = call "SEND_HEARTBEAT.vi"("error in (no error)"=w545) -> ("error out"=w544:errorcluster)  [unwired: 10 in]
    n166 = Subtract(x=w551, y=w550) -> (x-y=w549:dbl)
    n167 = Greater?(x=w549, y=2.0) -> (0:w547:bool)
    n168 = Not(x=w547) -> (.not. x?=w540:bool)
    n169 = call-poly <userlib>:"Data Changed__ogtk.vi"("Boolean"=w540) -> ("Changed"=w541:bool)
    n170 = case shown="False" w540 {
      frame False {
        n171 = feedback #1(TRUE) -> (w558:bool)
        n172 = Not(x=w558) -> (.not. x?=w557:bool)
        n173 = feedback-in #1(w557) -> ()
        n174 = Boolean To (0,1)(Boolean=w557) -> (0, 1=→"Connecting":i16)
      }
      frame True {
      }
    }
    n175 = case shown="True" w541 {
      tunnel: w544 -> [w560 w563]
      tunnel: [w560 w562] -> w543
      tunnel: w540 -> [_ w561]
      frame False {
        # "Sensor not connected fo go to waiting"
      }
      frame True {
        # "State Change"
        n176 = case shown="False" w561 {
          tunnel: w563 -> [w565 w568]
          tunnel: [w566 w567] -> w562
          frame False {
            n177 = call "Set Comms Loop Next State.vi"("Command"=Comms_Loop_States."Sensor Disconnected", "error in (no error)"=w565) -> ("error out"=w566:errorcluster)  [unwired: 9 in]
          }
          frame True {
            n178 = call "Set Comms Loop Next State.vi"("Command"=Comms_Loop_States."Sensor Connected", "error in (no error)"=w568) -> ("error out"=w567:errorcluster)  [unwired: 9 in]
          }
        }
      }
    }
    n179 = global write "Message Globals.vi" "Sensor Connected?"(w540) -> ()
    n180 = call-poly "Stop Button.vi"("Error In"=w543) -> ("Error Out"=w546:errorcluster, "Stop ButtonOut"=w542:bool)  [unwired: 9 in]
    n181 = Or(x=w546, y=w542) -> (x .or. y?=w555:bool)
    n182 = Wait (ms)(milliseconds to wait=u32 1000) -> ()  [unwired: 1 out]
  }
  n183 = Merge Errors(w13, w22, w12, w10) -> (w21:errorcluster)
  n184 = UDP Close(connection ID=w11, 8:w21) -> (error out=w23:errorcluster)  [unwired: 1 out]
  n185 = call <vilib>:"Simple Error Handler.vi"("error in (no error)"=w23) -> ()  [unwired: 4 in, 5 out]
